vi "FTW-TestStep-Base_TestExecInbox_Get.vi"(8 "error in (no error)":errorcluster, 11 "FTW-ScripterStep-Base in":refnum<class "FTW-TestStep-Base.lvclass">) -> (0 "error out":errorcluster, 2 "Scripter Inbox":string, 3 "FTW-ScripterStep-Base out":refnum<class "FTW-TestStep-Base.lvclass">)   [LabVIEW 2015, in "FTW-TestStep-Base.lvclass"]
uses:
  FTW-TestStep-Base.lvclass
  FTW-TestStep-Base.lvclass/FTW-TestStep-Base.ctl
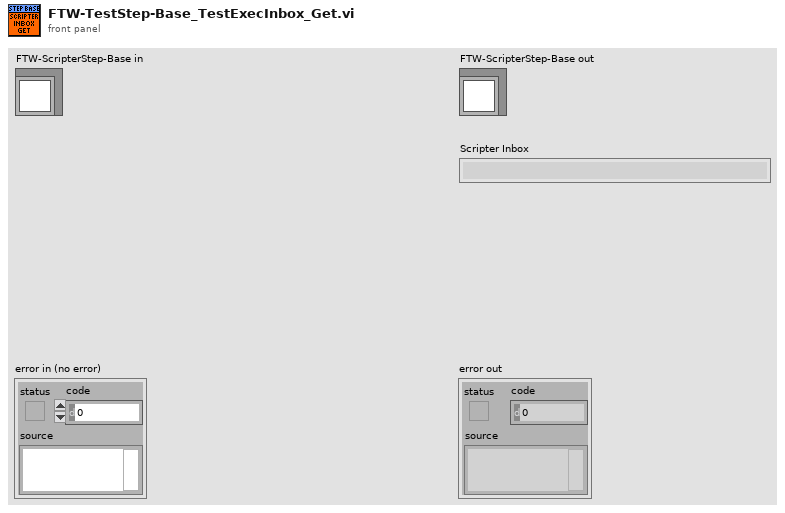
[diagram p1: front panel]
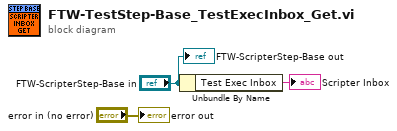
[diagram p0: block diagram]
diagram:
  n1 = Unbundle By Name("FTW-ScripterStep-Base in") -> ("Test Exec Inbox"=→"Scripter Inbox":string)
  "error out" <- "error in (no error)"
  "FTW-ScripterStep-Base out" <- "FTW-ScripterStep-Base in"
